vi "SW_Save_Settings.vi"() -> ()   [LabVIEW 2018]
uses:
  Controls/CTL_Settings_cluster.ctl
  Controls/CTL_Filter_selector.ctl
  Controls/CTL_Segmented_plot_parameters.ctl
  Controls/CTL_IO_params_cluster.ctl
  Controls/CTL_Single_stimulus_setting.ctl
  <vilib>/Utility/sysdir.llb/System Directory Type.ctl
  <vilib>/Utility/config.llb/NI_LVConfig.lvlib
panel:
  in  "Settings cluster in":T1={"Defaults"={"Default User"=0.0, "VISA Resource Name "=""}, "Recording and saving"={"Researcher name"="Researcher", "Name prefix"="Track", "Data filtering"={"Filter type"=enum."Savitzky-Golay", "Length"=31, "Order"=3}, "Stop at"=0.0, "\"Stop at\" enabled"=FALSE, "Default save folder path"=path ""}, "Geometry"={"Cage diameter, mm"=180, "Starting angle MIDFIELD"=0, "Starting angle BORDER"=0, "Radius, mm CENTER"=30, "Radius, mm MIDFIELD"=75, "N segments MIDFIELD"=2, "N segments BORDER"=4, "R-gap, mm"=0.0, "Bridge swap"=FALSE, "Bridge H. offset"=0.0, "Bridge V. offset"=0.0, "Twisted neck"=FALSE, "Alt. magn. orientation"=FALSE}, "IO parameters"={"IO general config."=12, "IO 1 configuration"=1, "IO 2 configuration"=1, "IO 3 configuration"=0, "IO 4 configuration"=0, "Activate ext. RS-232"=0, "IO inversion config."=0, "Sync capability"=1}, "Stimulus presets array"=[{"Event type"=0, "Dur., s"=0.0, "Stim., s"=0.0, "TTL out N"=1, "Set/Clear"=FALSE, "Stim. has been set"=FALSE}, {"Event type"=0, "Dur., s"=0.0, "Stim., s"=0.0, "TTL out N"=1, "Set/Clear"=FALSE, "Stim. has been set"=FALSE}, {"Event type"=0, "Dur., s"=0.0, "Stim., s"=0.0, "TTL out N"=1, "Set/Clear"=FALSE, "Stim. has been set"=FALSE}, {"Event type"=0, "Dur., s"=0.0, "Stim., s"=0.0, "TTL out N"=1, "Set/Clear"=FALSE, "Stim. has been set"=FALSE}, {"Event type"=0, "Dur., s"=0.0, "Stim., s"=0.0, "TTL out N"=1, "Set/Clear"=FALSE, "Stim. has been set"=FALSE}, {"Event type"=0, "Dur., s"=0.0, "Stim., s"=0.0, "TTL out N"=1, "Set/Clear"=FALSE, "Stim. has been set"=FALSE}, {"Event type"=0, "Dur., s"=0.0, "Stim., s"=0.0, "TTL out N"=1, "Set/Clear"=FALSE, "Stim. has been set"=FALSE}, {"Event type"=0, "Dur., s"=0.0, "Stim., s"=0.0, "TTL out N"=1, "Set/Clear"=FALSE, "Stim. has been set"=FALSE}, {"Event type"=0, "Dur., s"=0.0, "Stim., s"=0.0, "TTL out N"=1, "Set/Clear"=FALSE, "Stim. has been set"=FALSE}, {"Event type"=0, "Dur., s"=0.0, "Stim., s"=0.0, "TTL out N"=1, "Set/Clear"=FALSE, "Stim. has been set"=FALSE}, {"Event type"=0, "Dur., s"=0.0, "Stim., s"=0.0, "TTL out N"=1, "Set/Clear"=FALSE, "Stim. has been set"=FALSE}, {"Event type"=0, "Dur., s"=0.0, "Stim., s"=0.0, "TTL out N"=1, "Set/Clear"=FALSE, "Stim. has been set"=FALSE}, {"Event type"=0, "Dur., s"=0.0, "Stim., s"=0.0, "TTL out N"=1, "Set/Clear"=FALSE, "Stim. has been set"=FALSE}, {"Event type"=0, "Dur., s"=0.0, "Stim., s"=0.0, "TTL out N"=1, "Set/Clear"=FALSE, "Stim. has been set"=FALSE}], "Settings loaded OK"=FALSE} {"Stimulus presets array"."Event type" items=["Stay for N seconds"]; "Stimulus presets array"."TTL out N" items=["1"=1, "2"=2, "1+2"=3]; "Recording and saving"."Data filtering"."Order" min=3 max=11 step=2; "Recording and saving"."Data filtering"."Length" min=5 max=301 step=2; "Geometry"."Cage diameter, mm" scale=0.0..340.0}
  in  "Setting to Save":string(combo)
  out "Settings file path":path
  in  "Researcher name":string="Researcher"
  in  "Settings path in":path
  out "Settings cluster out":T1={"Defaults"={"Default User"=0.0, "VISA Resource Name "=""}, "Recording and saving"={"Researcher name"="", "Name prefix"="", "Data filtering"={"Filter type"=enum."Savitzky-Golay", "Length"=31, "Order"=3}, "Stop at"=0.0, "\"Stop at\" enabled"=FALSE, "Default save folder path"=path ""}, "Geometry"={"Cage diameter, mm"=0, "Starting angle MIDFIELD"=0, "Starting angle BORDER"=0, "Radius, mm CENTER"=0, "Radius, mm MIDFIELD"=0, "N segments MIDFIELD"=0, "N segments BORDER"=0, "R-gap, mm"=0.0, "Bridge swap"=FALSE, "Bridge H. offset"=0.0, "Bridge V. offset"=0.0, "Twisted neck"=FALSE, "Alt. magn. orientation"=FALSE}, "IO parameters"={"IO general config."=0, "IO 1 configuration"=0, "IO 2 configuration"=0, "IO 3 configuration"=0, "IO 4 configuration"=0, "Activate ext. RS-232"=0, "IO inversion config."=0, "Sync capability"=1}, "Stimulus presets array"=[{"Event type"=0, "Dur., s"=0.0, "Stim., s"=0.0, "TTL out N"=1, "Set/Clear"=FALSE, "Stim. has been set"=FALSE}, {"Event type"=0, "Dur., s"=0.0, "Stim., s"=0.0, "TTL out N"=1, "Set/Clear"=FALSE, "Stim. has been set"=FALSE}, {"Event type"=0, "Dur., s"=0.0, "Stim., s"=0.0, "TTL out N"=1, "Set/Clear"=FALSE, "Stim. has been set"=FALSE}, {"Event type"=0, "Dur., s"=0.0, "Stim., s"=0.0, "TTL out N"=1, "Set/Clear"=FALSE, "Stim. has been set"=FALSE}, {"Event type"=0, "Dur., s"=0.0, "Stim., s"=0.0, "TTL out N"=1, "Set/Clear"=FALSE, "Stim. has been set"=FALSE}, {"Event type"=0, "Dur., s"=0.0, "Stim., s"=0.0, "TTL out N"=1, "Set/Clear"=FALSE, "Stim. has been set"=FALSE}, {"Event type"=0, "Dur., s"=0.0, "Stim., s"=0.0, "TTL out N"=1, "Set/Clear"=FALSE, "Stim. has been set"=FALSE}, {"Event type"=0, "Dur., s"=0.0, "Stim., s"=0.0, "TTL out N"=1, "Set/Clear"=FALSE, "Stim. has been set"=FALSE}, {"Event type"=0, "Dur., s"=0.0, "Stim., s"=0.0, "TTL out N"=1, "Set/Clear"=FALSE, "Stim. has been set"=FALSE}, {"Event type"=0, "Dur., s"=0.0, "Stim., s"=0.0, "TTL out N"=1, "Set/Clear"=FALSE, "Stim. has been set"=FALSE}, {"Event type"=0, "Dur., s"=0.0, "Stim., s"=0.0, "TTL out N"=1, "Set/Clear"=FALSE, "Stim. has been set"=FALSE}, {"Event type"=0, "Dur., s"=0.0, "Stim., s"=0.0, "TTL out N"=1, "Set/Clear"=FALSE, "Stim. has been set"=FALSE}, {"Event type"=0, "Dur., s"=0.0, "Stim., s"=0.0, "TTL out N"=1, "Set/Clear"=FALSE, "Stim. has been set"=FALSE}, {"Event type"=0, "Dur., s"=0.0, "Stim., s"=0.0, "TTL out N"=1, "Set/Clear"=FALSE, "Stim. has been set"=FALSE}], "Settings loaded OK"=FALSE} {"Stimulus presets array"."Event type" items=["Stay for N seconds"]; "Stimulus presets array"."TTL out N" items=["1"=1, "2"=2, "1+2"=3]; "Recording and saving"."Data filtering"."Order" min=3 max=11 step=2; "Recording and saving"."Data filtering"."Length" min=5 max=301 step=2; "Geometry"."Cage diameter, mm" scale=0.0..340.0}
  in  "error in (no error)":errorcluster
  out "error out":errorcluster={"status"=TRUE, "code"=1, "source"="Dequeue Element in NI_LVConfig.lvlib:Read Value Without Comment.vi->NI_LVConfig.lvlib:Read Key (I32).vi->SW_Load_settings_to_main_tab.vi"}
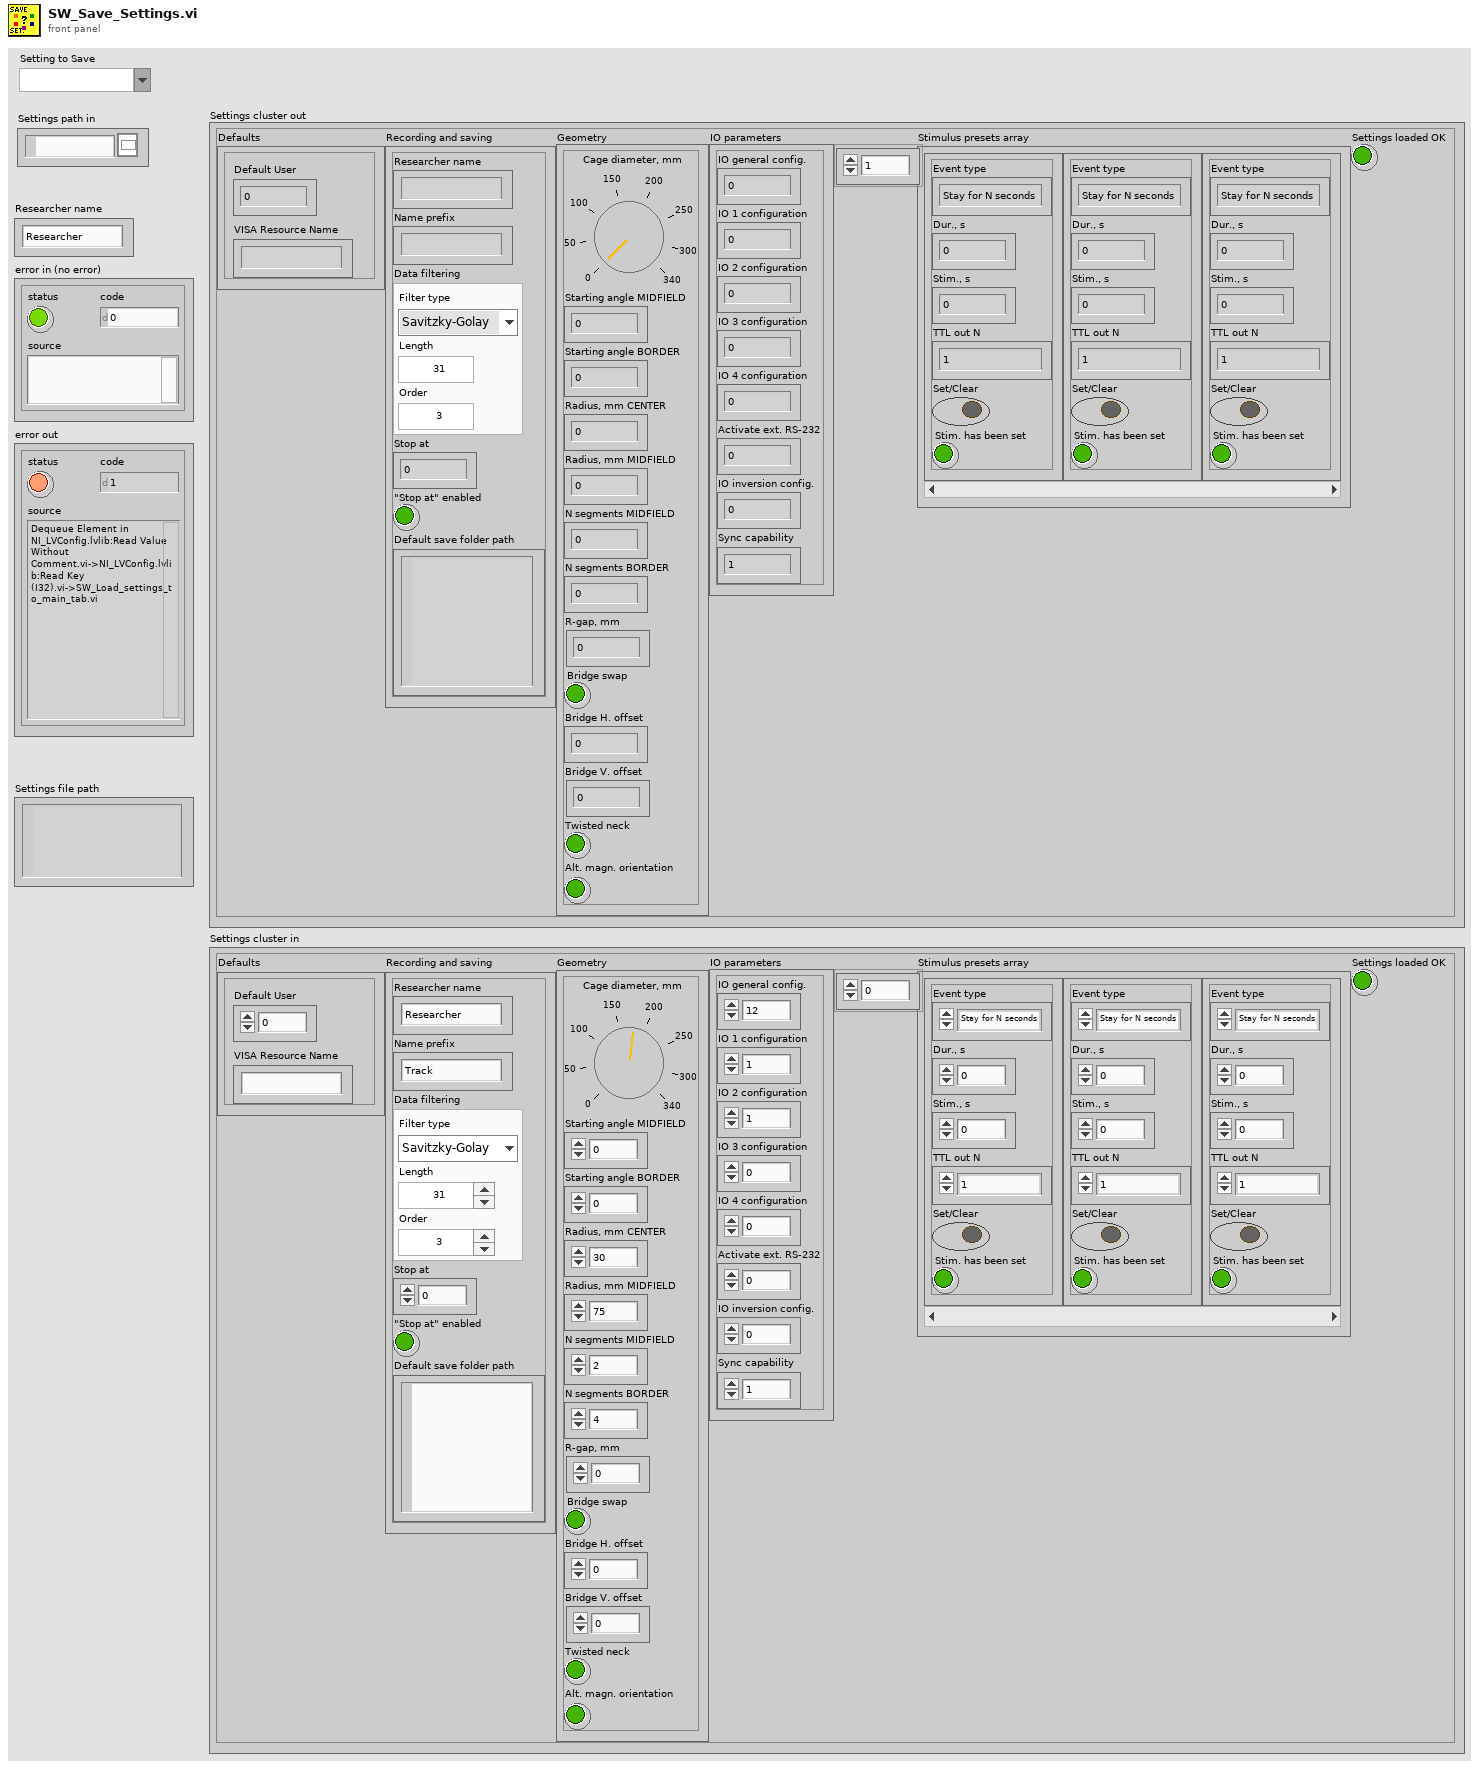
[diagram p1: front panel]
types:
  T1 = typedef "CTL_Settings_cluster.ctl" = cluster{"Defaults":cluster{"Default User":dbl, "VISA Resource Name ":string}, "Recording and saving":cluster{"Researcher name":string, "Name prefix":string, "Data filtering":T2, "Stop at":dbl, "\"Stop at\" enabled":bool, "Default save folder path":path}, "Geometry":T3, "IO parameters":T4, "Stimulus presets array":T5[], "Settings loaded OK":bool}
  T2 = typedef "CTL_Filter_selector.ctl" = cluster{"Filter type":enum16{"None", "Savitzky-Golay"}, "Length":i32, "Order":i32}
  T3 = typedef "CTL_Segmented_plot_parameters.ctl" = cluster{"Cage diameter, mm":u16, "Starting angle MIDFIELD":i16, "Starting angle BORDER":i16, "Radius, mm CENTER":u16, "Radius, mm MIDFIELD":u16, "N segments MIDFIELD":u8, "N segments BORDER":u8, "R-gap, mm":sgl, "Bridge swap":bool, "Bridge H. offset":sgl, "Bridge V. offset":sgl, "Twisted neck":bool, "Alt. magn. orientation":bool}
  T4 = typedef "CTL_IO_params_cluster.ctl" = cluster{"IO general config.":u16, "IO 1 configuration":u16, "IO 2 configuration":u16, "IO 3 configuration":u16, "IO 4 configuration":u16, "Activate ext. RS-232":u16, "IO inversion config.":u16, "Sync capability":u8}
  T5 = typedef "CTL_Single_stimulus_setting.ctl" = cluster{"Event type":u16, "Dur., s":sgl, "Stim., s":sgl, "TTL out N":u16, "Set/Clear":bool, "Stim. has been set":bool}
  T6 = typedef "NI_LVConfig.lvlib/Config Data RefNum.ctl" = refnum<k1>
  T7 = cluster{"Default User":dbl, "VISA Resource Name ":string}
  T8 = cluster{"Researcher name":string, "Name prefix":string, "Data filtering":T2, "Stop at":dbl, "\"Stop at\" enabled":bool, "Default save folder path":path}
  T9 = typedef "System Directory Type.ctl" = i32
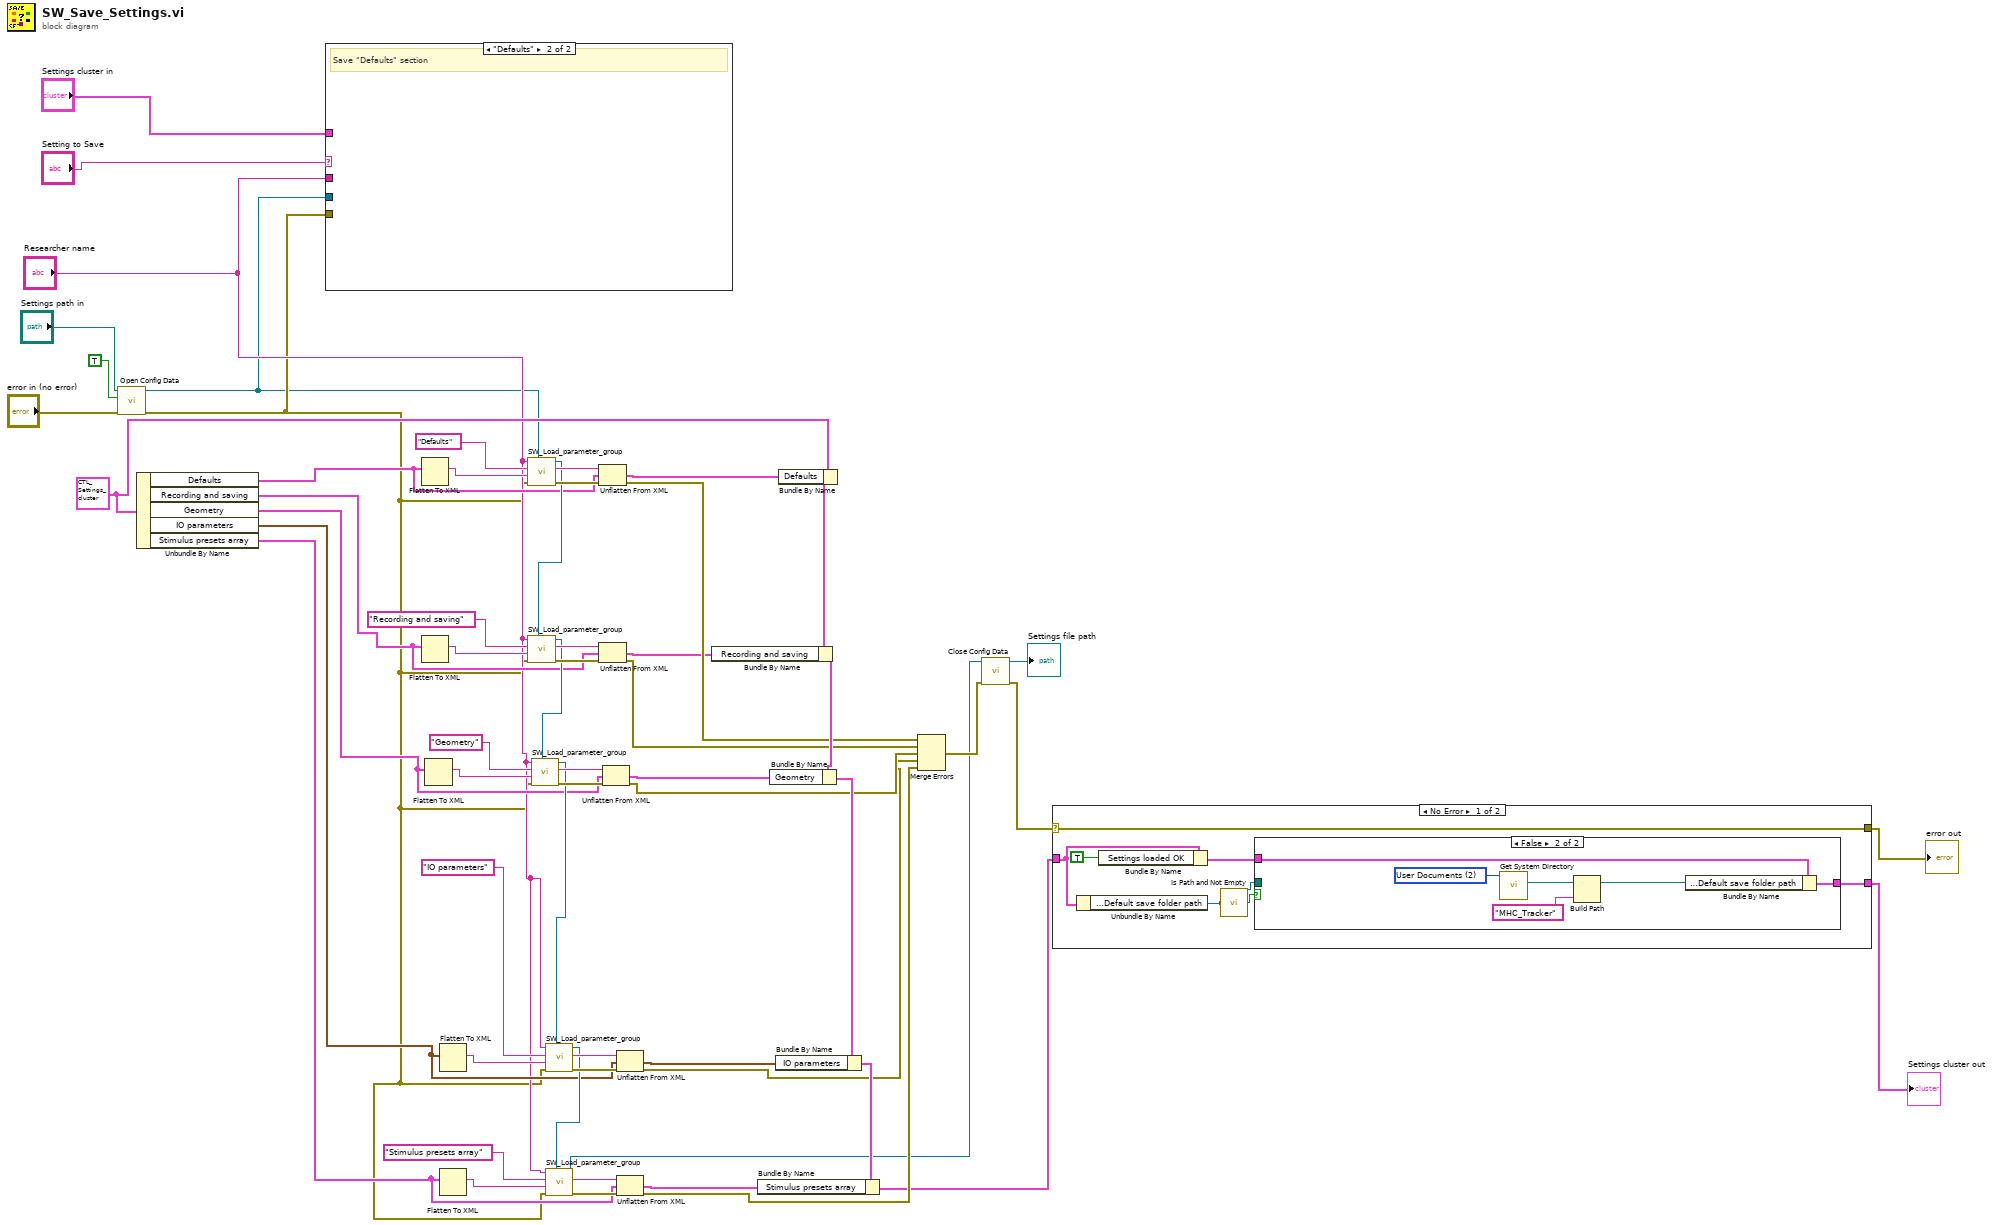
[diagram p0: block diagram]
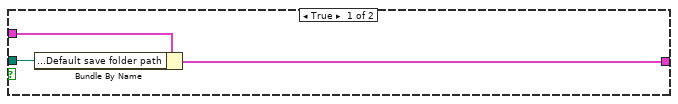
[diagram p3: hidden frame]
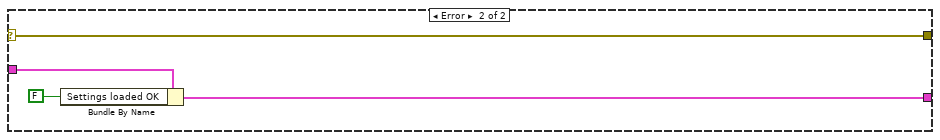
[diagram p4: hidden frame]
diagram:
  w40 = T1 {"Defaults"={"Default User"=0.0, "VISA Resource Name "=""}, "Recording and saving"={"Researcher name"="Researcher", "Name prefix"="Track", "Data filtering"={"Filter type"=enum."Savitzky-Golay", "Length"=31, "Order"=3}, "Stop at"=0.0, "\"Stop at\" enabled"=FALSE, "Default save folder path"=path ""}, "Geometry"={"Cage diameter, mm"=180, "Starting angle MIDFIELD"=0, "Starting angle BORDER"=0, "Radius, mm CENTER"=30, "Radius, mm MIDFIELD"=75, "N segments MIDFIELD"=2, "N segments BORDER"=4, "R-gap, mm"=0.0, "Bridge swap"=FALSE, "Bridge H. offset"=0.0, "Bridge V. offset"=0.0, "Twisted neck"=FALSE, "Alt. magn. orientation"=FALSE}, "IO parameters"={"IO general config."=12, "IO 1 configuration"=1, "IO 2 configuration"=1, "IO 3 configuration"=0, "IO 4 configuration"=0, "Activate ext. RS-232"=0, "IO inversion config."=0, "Sync capability"=1}, "Stimulus presets array"=[{"Event type"=0, "Dur., s"=0.0, "Stim., s"=0.0, "TTL out N"=1, "Set/Clear"=FALSE, "Stim. has been set"=FALSE}, {"Event type"=0, "Dur., s"=0.0, "Stim., s"=0.0, "TTL out N"=1, "Set/Clear"=FALSE, "Stim. has been set"=FALSE}, {"Event type"=0, "Dur., s"=0.0, "Stim., s"=0.0, "TTL out N"=1, "Set/Clear"=FALSE, "Stim. has been set"=FALSE}, {"Event type"=0, "Dur., s"=0.0, "Stim., s"=0.0, "TTL out N"=1, "Set/Clear"=FALSE, "Stim. has been set"=FALSE}, {"Event type"=0, "Dur., s"=0.0, "Stim., s"=0.0, "TTL out N"=1, "Set/Clear"=FALSE, "Stim. has been set"=FALSE}, {"Event type"=0, "Dur., s"=0.0, "Stim., s"=0.0, "TTL out N"=1, "Set/Clear"=FALSE, "Stim. has been set"=FALSE}, {"Event type"=0, "Dur., s"=0.0, "Stim., s"=0.0, "TTL out N"=1, "Set/Clear"=FALSE, "Stim. has been set"=FALSE}, {"Event type"=0, "Dur., s"=0.0, "Stim., s"=0.0, "TTL out N"=1, "Set/Clear"=FALSE, "Stim. has been set"=FALSE}, {"Event type"=0, "Dur., s"=0.0, "Stim., s"=0.0, "TTL out N"=1, "Set/Clear"=FALSE, "Stim. has been set"=FALSE}, {"Event type"=0, "Dur., s"=0.0, "Stim., s"=0.0, "TTL out N"=1, "Set/Clear"=FALSE, "Stim. has been set"=FALSE}, {"Event type"=0, "Dur., s"=0.0, "Stim., s"=0.0, "TTL out N"=1, "Set/Clear"=FALSE, "Stim. has been set"=FALSE}, {"Event type"=0, "Dur., s"=0.0, "Stim., s"=0.0, "TTL out N"=1, "Set/Clear"=FALSE, "Stim. has been set"=FALSE}, {"Event type"=0, "Dur., s"=0.0, "Stim., s"=0.0, "TTL out N"=1, "Set/Clear"=FALSE, "Stim. has been set"=FALSE}, {"Event type"=0, "Dur., s"=0.0, "Stim., s"=0.0, "TTL out N"=1, "Set/Clear"=FALSE, "Stim. has been set"=FALSE}], "Settings loaded OK"=FALSE} ("Settings cluster")
  n1 = call <vilib>:"Open Config Data.vi"("error in (no error)"="error in (no error)", "create file if necessary (T)"=TRUE, "configuration file path"="Settings path in") -> ("error out"=w3:errorcluster, "refnum"=w1:T6)  [unwired: 6 in, 1 out]
  n2 = Unbundle By Name(w40) -> ("Defaults"=w6:T7, "Recording and saving"=w7:T8, "Geometry"=w31:T3, "IO parameters"=w11:T4, "Stimulus presets array"=w10:T5[])
  n3 = case shown="\"Defaults\"" "Setting to Save" {
    tunnel: "Researcher name" -> [_ _]
    tunnel: w3 -> [_ _]
    tunnel: "Settings cluster in" -> [_ _]
    tunnel: w1 -> [_ _]
    frame "\u0000", Default {
    }
    frame "Defaults" {
      # "Save \"Defaults\" section"
    }
  }
  n4 = Flatten To XML(anything=w6) -> (xml string=w55:string)
  n5 = Flatten To XML(anything=w7) -> (xml string=w49:string)
  n6 = Flatten To XML(anything=w31) -> (xml string=w45:string)
  n7 = Flatten To XML(anything=w11) -> (xml string=w34:string)
  n8 = Flatten To XML(anything=w10) -> (xml string=w28:string)
  n9 = call "SW_Load_parameter_group.vi"("Settings file refnum in"=w1, "error in"=w3, "Default value"=w55, "Param group"="Defaults" ("Group"), "Researcher name"="Researcher name") -> ("error out"=w56:errorcluster, "Read value"=w53:string, "Settings file refnum out"=w47:T6)  [unwired: 4 in]
  n10 = call "SW_Load_parameter_group.vi"("Settings file refnum in"=w47, "error in"=w3, "Default value"=w49, "Param group"="Recording and saving" ("Group"), "Researcher name"="Researcher name") -> ("error out"=w48:errorcluster, "Read value"=w51:string, "Settings file refnum out"=w41:T6)  [unwired: 4 in]
  n11 = call "SW_Load_parameter_group.vi"("Settings file refnum in"=w41, "error in"=w3, "Default value"=w45, "Param group"="Geometry" ("Group"), "Researcher name"="Researcher name") -> ("error out"=w46:errorcluster, "Read value"=w43:string, "Settings file refnum out"=w32:T6)  [unwired: 4 in]
  n12 = call "SW_Load_parameter_group.vi"("Settings file refnum in"=w32, "error in"=w3, "Default value"=w34, "Param group"="IO parameters" ("Group"), "Researcher name"="Researcher name") -> ("error out"=w33:errorcluster, "Read value"=w36:string, "Settings file refnum out"=w23:T6)  [unwired: 4 in]
  n13 = call "SW_Load_parameter_group.vi"("Settings file refnum in"=w23, "error in"=w3, "Default value"=w28, "Param group"="Stimulus presets array" ("Group"), "Researcher name"="Researcher name") -> ("error out"=w29:errorcluster, "Read value"=w26:string, "Settings file refnum out"=w8:T6)  [unwired: 4 in]
  n14 = Unflatten From XML(xml string=w53, type=w6, error in (no error)=w56) -> (value=w52:T7, error out=w22:errorcluster)
  n15 = Unflatten From XML(xml string=w51, type=w7, error in (no error)=w48) -> (value=w13:T8, error out=w21:errorcluster)
  n16 = Unflatten From XML(xml string=w43, type=w31, error in (no error)=w46) -> (value=w42:T3, error out=w20:errorcluster)
  n17 = Unflatten From XML(xml string=w36, type=w11, error in (no error)=w33) -> (value=w37:T4, error out=w19:errorcluster)
  n18 = Unflatten From XML(xml string=w26, type=w10, error in (no error)=w29) -> (value=w25:T5[], error out=w18:errorcluster)
  n19 = Bundle By Name(cluster=w40, "Defaults"=w52) -> (w39:T1)
  n20 = Bundle By Name(cluster=w39, "Recording and saving"=w13) -> (w38:T1)
  n21 = Bundle By Name(cluster=w38, "Geometry"=w42) -> (w30:T1)
  n22 = Bundle By Name(cluster=w30, "IO parameters"=w37) -> (w24:T1)
  n23 = Bundle By Name(cluster=w24, "Stimulus presets array"=w25) -> (w9:T1)
  n24 = Merge Errors(w22, w21, w20, w19, w18) -> (w17:errorcluster)
  n25 = call <vilib>:"Close Config Data.vi"("error in (no error)"=w17, "refnum"=w8) -> ("error out"=w16:errorcluster, "file path"=→"Settings file path":path)  [unwired: 8 in]
  n26 = case shown="No Error" w16 {
    selector: w16 -> [w65 w77]
    tunnel: [w65 w77] -> w15
    tunnel: w9 -> [w64 w79]
    tunnel: [w60 w76] -> w14
    frame No Error {
      n27 = Unbundle By Name(w64) -> ("Recording and saving.Default save folder path"=w61:path)
      n28 = Bundle By Name(cluster=w64, "Settings loaded OK"=TRUE) -> (w62:T1)
      n29 = call <vilib>:"Is Path and Not Empty.vi"("path"=w61) -> ("Is Path and Not Empty?"=w63:bool)  [unwired: 4 in]
      n30 = case shown="False" w63 {
        tunnel: w62 -> [w69 w75]
        tunnel: w61 -> [w68 _]
        tunnel: [w67 w74] -> w60
        frame True {
          n31 = Bundle By Name(cluster=w69, "Recording and saving.Default save folder path"=w68) -> (w67:T1)
        }
        frame False {
          w72 = T9 2 items=["User Home"=0, "User Desktop"=1, "User Documents"=2, "User Application Data"=3, "User Preferences"=4, "User Temporary"=5, "Public Documents"=6, "Public Application Data"=7, "Public Preferences"=8, "Public Cache"=13, "System Core Libraries"=9, "System Installed Libraries"=10, "Application Files"=11, "Boot Volume Root"=12] ("system directory type")
          n32 = call <vilib>:"Get System Directory.vi"("system directory type"=w72) -> ("system directory"=w73:path)  [unwired: 10 in]
          n33 = Build Path(base path=w73, name or relative path="MHC_Tracker") -> (appended path=w71:path)
          n34 = Bundle By Name(cluster=w75, "Recording and saving.Default save folder path"=w71) -> (w74:T1)
        }
      }
    }
    frame Error {
      n35 = Bundle By Name(cluster=w79, "Settings loaded OK"=FALSE) -> (w76:T1)
    }
  }
  "Settings cluster out" <- w14
  "error out" <- w15
